vi "Left Motor Control Loop (SubVI).vi"   [LabVIEW 2015]
uses:
  Left Variables.vi
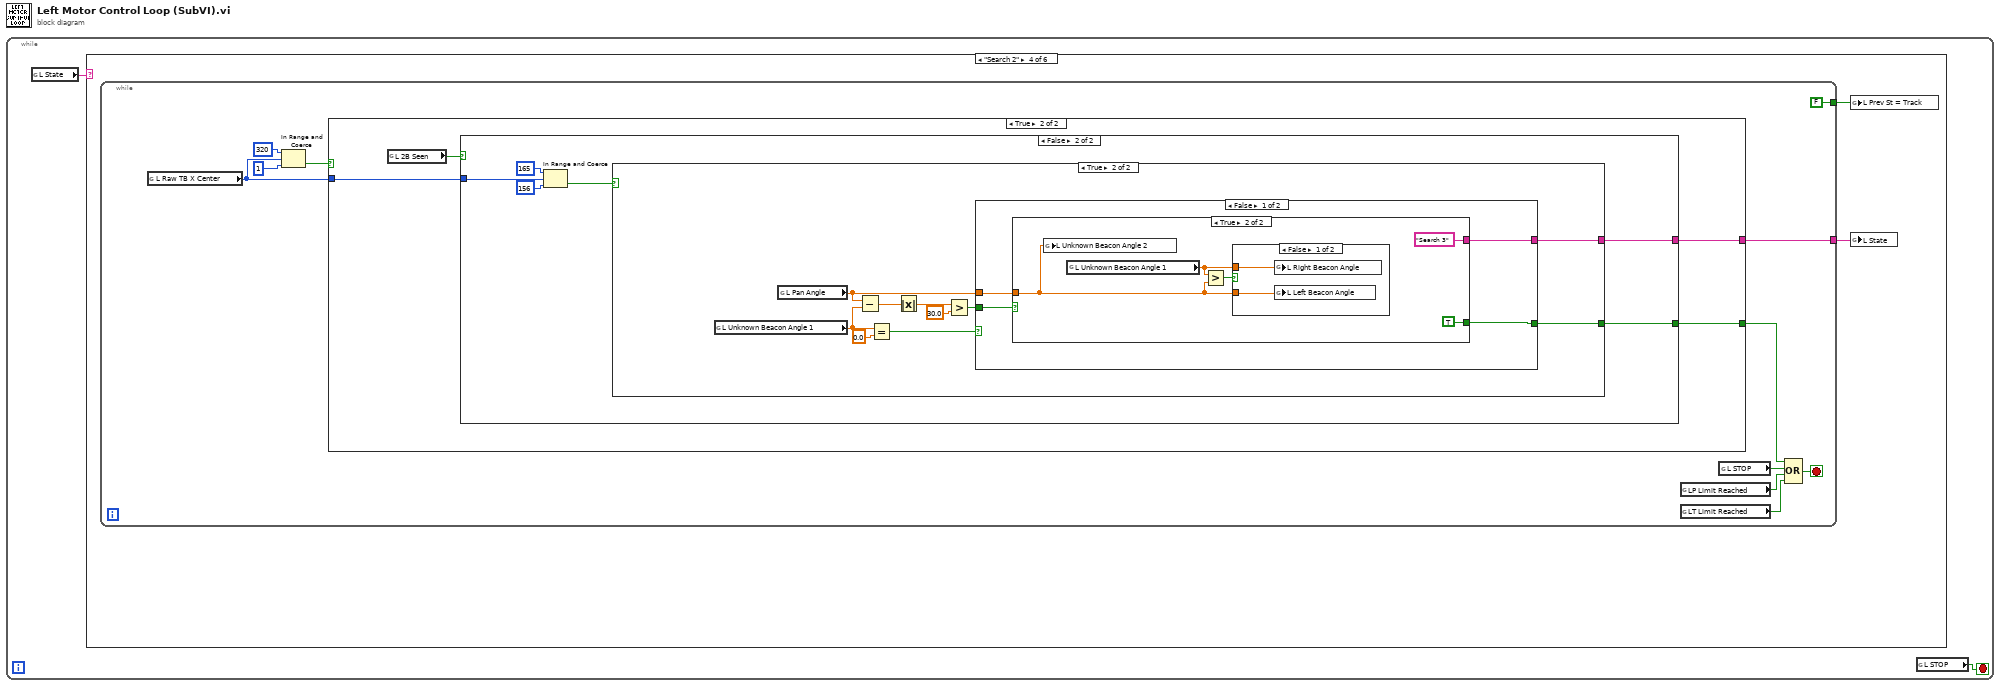
[diagram p0: block diagram]
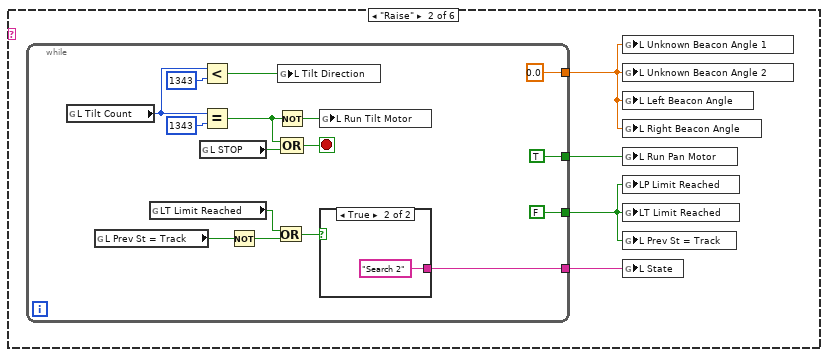
[diagram p3: hidden frame]
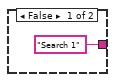
[diagram p4: hidden frame]
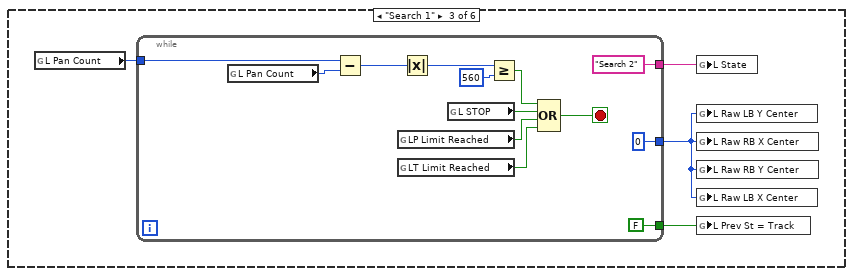
[diagram p5: hidden frame]
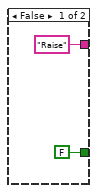
[diagram p6: hidden frame]
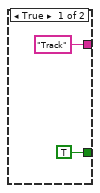
[diagram p7: hidden frame]
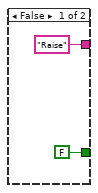
[diagram p8: hidden frame]
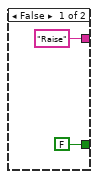
[diagram p9: hidden frame]
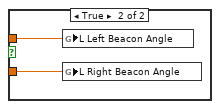
[diagram p10: hidden frame]
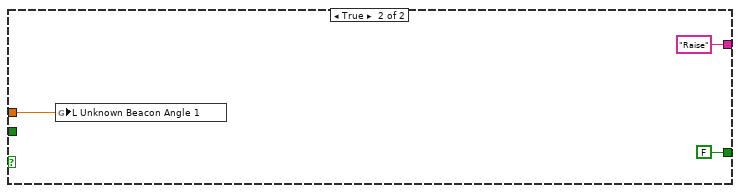
[diagram p11: hidden frame]
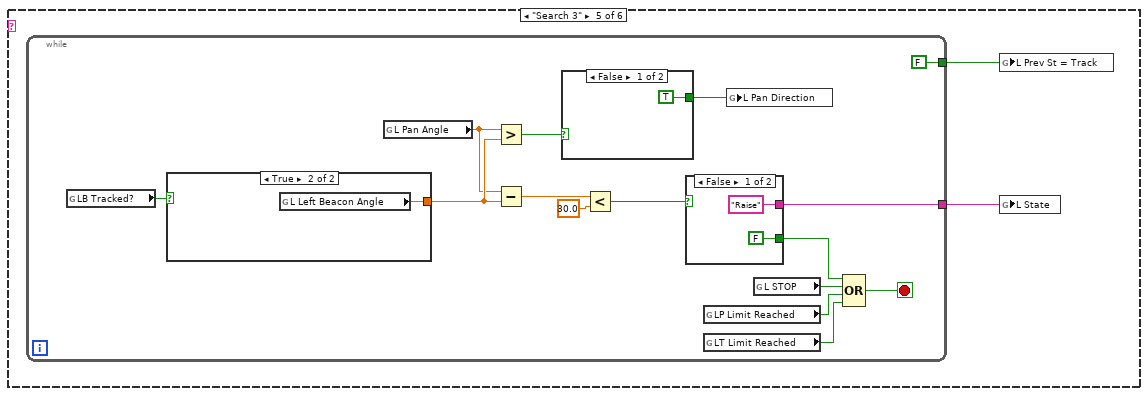
[diagram p12: hidden frame]
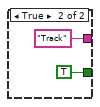
[diagram p13: hidden frame]
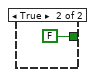
[diagram p14: hidden frame]
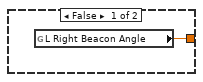
[diagram p15: hidden frame]
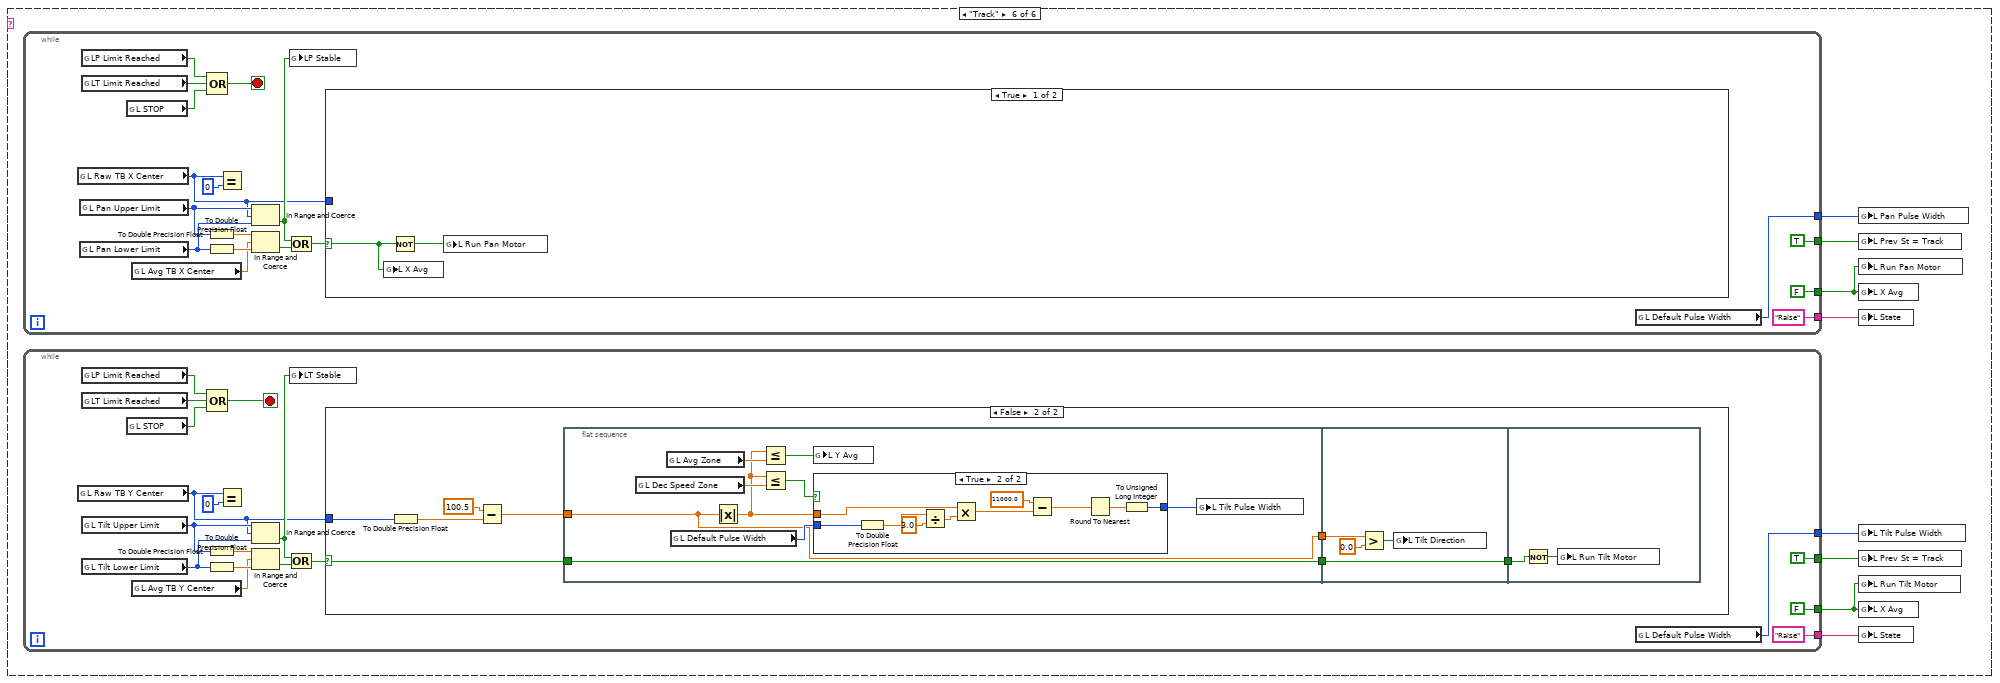
[diagram p16: hidden frame]
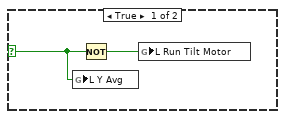
[diagram p17: hidden frame]
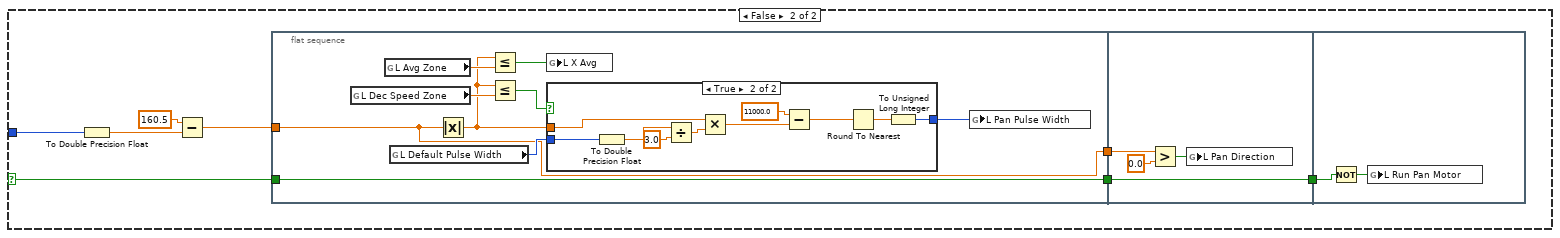
[diagram p19: hidden frame]
diagram:
  n1 = while {
    stop <- w1 stop-if-true
    n2 = global read "Left Variables.vi" "L State"() -> (w2:string)
    n3 = case shown="\"Search 2\"" w2 {
      frame "Null", Default {
      }
      frame "Raise" {
        n4 = while {
          tunnel: [w14] -> w6
          tunnel: [FALSE ("y")] -> w3
          tunnel: [TRUE ("y")] -> w5
          tunnel: [0.0] -> w4
          stop <- w22 stop-if-true
          n5 = global read "Left Variables.vi" "L Tilt Count"() -> (w18:i32)
          n6 = global read "Left Variables.vi" "L Prev St = Track"() -> (w10:bool)
          n7 = global read "Left Variables.vi" "LT Limit Reached"() -> (w8:bool)
          n8 = global read "Left Variables.vi" "L STOP"() -> (w15:bool)
          n9 = Less?(x=w18, y=1343) -> (x < y?=w20:bool)
          n10 = Equal?(x=w18, y=1343) -> (x = y?=w16:bool)
          n11 = Not(x=w10) -> (.not. x?=w9:bool)
          n12 = Or(x=w8, y=w9) -> (x .or. y?=w7:bool)
          n13 = Not(x=w16) -> (.not. x?=w17:bool)
          n14 = global write "Left Variables.vi" "L Tilt Direction"(w20) -> ()
          n15 = Compound Arithmetic op=OR(w16, w15) -> (w22:bool)
          n16 = global write "Left Variables.vi" "L Run Tilt Motor"(w17) -> ()
          n17 = case shown="True" w7 {
            tunnel: ["Search 1" ("L State") "Search 2" ("L State")] -> w14
            frame False {
            }
            frame True {
            }
          }
        }
        n18 = global write "Left Variables.vi" "L Unknown Beacon Angle 1"(w4) -> ()
        n19 = global write "Left Variables.vi" "L Unknown Beacon Angle 2"(w4) -> ()
        n20 = global write "Left Variables.vi" "L Left Beacon Angle"(w4) -> ()
        n21 = global write "Left Variables.vi" "L Right Beacon Angle"(w4) -> ()
        n22 = global write "Left Variables.vi" "L Run Pan Motor"(w5) -> ()
        n23 = global write "Left Variables.vi" "LP Limit Reached"(w3) -> ()
        n24 = global write "Left Variables.vi" "LT Limit Reached"(w3) -> ()
        n25 = global write "Left Variables.vi" "L Prev St = Track"(w3) -> ()
        n26 = global write "Left Variables.vi" "L State"(w6) -> ()
      }
      frame "Search 1" {
        n27 = global read "Left Variables.vi" "L Pan Count"() -> (w27:i32)
        n28 = while {
          tunnel: ["Search 2"] -> w28
          tunnel: w27 -> [w37]
          tunnel: [u16 0] -> w26
          tunnel: [FALSE] -> w25
          stop <- w41 stop-if-true
          n29 = global read "Left Variables.vi" "L Pan Count"() -> (w34:i32)
          n30 = Subtract(x=w37, y=w34) -> (x-y=w36:i32)
          n31 = global read "Left Variables.vi" "LP Limit Reached"() -> (w31:bool)
          n32 = global read "Left Variables.vi" "LT Limit Reached"() -> (w30:bool)
          n33 = Absolute Value(x=w36) -> (abs(x)=w35:i32)
          n34 = global read "Left Variables.vi" "L STOP"() -> (w33:bool)
          n35 = Greater Or Equal?(x=w35, y=560) -> (x >= y?=w38:bool)
          n36 = Compound Arithmetic op=OR(w38, w33, w31, w30) -> (w41:bool)
        }
        n37 = global write "Left Variables.vi" "L State"(w28) -> ()
        n38 = global write "Left Variables.vi" "L Raw LB Y Center"(w26) -> ()
        n39 = global write "Left Variables.vi" "L Raw RB X Center"(w26) -> ()
        n40 = global write "Left Variables.vi" "L Raw RB Y Center"(w26) -> ()
        n41 = global write "Left Variables.vi" "L Raw LB X Center"(w26) -> ()
        n42 = global write "Left Variables.vi" "L Prev St = Track"(w25) -> ()
      }
      frame "Search 2" {
        n43 = while {
          tunnel: [w49] -> w43
          tunnel: [FALSE] -> w42
          stop <- w51 stop-if-true
          n44 = global read "Left Variables.vi" "L Raw TB X Center"() -> (w47:u16)
          n45 = In Range and Coerce(upper limit=u16 320, x=w47, lower limit=u16 1) -> (In Range?=w50:bool)  [unwired: 1 out]
          n46 = case shown="True" w50 {
            tunnel: [FALSE w60] -> w48
            tunnel: ["Raise" w59] -> w49
            tunnel: w47 -> [_ w58]
            frame False {
            }
            frame True {
              n47 = global read "Left Variables.vi" "L 2B Seen"() -> (w57:bool)
              n48 = case shown="False" w57 {
                tunnel: [TRUE w65] -> w60
                tunnel: ["Track" w64] -> w59
                tunnel: w58 -> [_ w63]
                frame True {
                }
                frame False {
                  n49 = In Range and Coerce(upper limit=u16 165, x=w63, lower limit=u16 156) -> (In Range?=w66:bool)  [unwired: 1 out]
                  n50 = case shown="True" w66 {
                    tunnel: [FALSE w73] -> w65
                    tunnel: ["Raise" w72] -> w64
                    frame False {
                    }
                    frame True {
                      n51 = global read "Left Variables.vi" "L Unknown Beacon Angle 1"() -> (w79:dbl)
                      n52 = global read "Left Variables.vi" "L Pan Angle"() -> (w71:dbl)
                      n53 = Subtract(x=w71, y=w79) -> (x-y=w78:dbl)
                      n54 = Equal?(x=w79, y=0.0) -> (x = y?=w75:bool)
                      n55 = Absolute Value(x=w78) -> (abs(x)=w77:dbl)
                      n56 = Greater?(x=w77, y=30.0) -> (0:w74:bool)
                      n57 = case shown="False" w75 {
                        tunnel: w71 -> [w84 w98]
                        tunnel: w74 -> [w83 _]
                        tunnel: [w82 FALSE] -> w73
                        tunnel: [w81 "Raise"] -> w72
                        frame False {
                          n58 = case shown="True" w83 {
                            tunnel: w84 -> [_ w87]
                            tunnel: [FALSE TRUE] -> w82
                            tunnel: ["Raise" "Search 3"] -> w81
                            frame False {
                            }
                            frame True {
                              n59 = global write "Left Variables.vi" "L Unknown Beacon Angle 2"(w87) -> ()
                              n60 = global read "Left Variables.vi" "L Unknown Beacon Angle 1"() -> (w90:dbl)
                              n61 = Greater?(x=w90, y=w87) -> (0:w91:bool)
                              n62 = case shown="False" w91 {
                                tunnel: w90 -> [w93 w95]
                                tunnel: w87 -> [w92 w94]
                                frame False {
                                n63 = global write "Left Variables.vi" "L Right Beacon Angle"(w93) -> ()
                                n64 = global write "Left Variables.vi" "L Left Beacon Angle"(w92) -> ()
                                }
                                frame True {
                                n65 = global write "Left Variables.vi" "L Left Beacon Angle"(w95) -> ()
                                n66 = global write "Left Variables.vi" "L Right Beacon Angle"(w94) -> ()
                                }
                              }
                            }
                          }
                        }
                        frame True {
                          n67 = global write "Left Variables.vi" "L Unknown Beacon Angle 1"(w98) -> ()
                        }
                      }
                    }
                  }
                }
              }
            }
          }
          n68 = global read "Left Variables.vi" "LP Limit Reached"() -> (w46:bool)
          n69 = global read "Left Variables.vi" "LT Limit Reached"() -> (w45:bool)
          n70 = global read "Left Variables.vi" "L STOP"() -> (w52:bool)
          n71 = Compound Arithmetic op=OR(w48, w52, w46, w45) -> (w51:bool)
        }
        n72 = global write "Left Variables.vi" "L Prev St = Track"(w42) -> ()
        n73 = global write "Left Variables.vi" "L State"(w43) -> ()
      }
      frame "Search 3" {
        n74 = while {
          tunnel: [w102] -> w100
          tunnel: [FALSE] -> w99
          stop <- w109 stop-if-true
          n75 = global read "Left Variables.vi" "LB Tracked?"() -> (w108:bool)
          n76 = case shown="True" w108 {
            tunnel: [w122 w123] -> w114
            frame False {
              n77 = global read "Left Variables.vi" "L Right Beacon Angle"() -> (w122:dbl)
            }
            frame True {
              n78 = global read "Left Variables.vi" "L Left Beacon Angle"() -> (w123:dbl)
            }
          }
          n79 = global read "Left Variables.vi" "L Pan Angle"() -> (w106:dbl)
          n80 = Greater?(x=w106, y=w114) -> (0:w115:bool)
          n81 = Subtract(x=w106, y=w114) -> (x-y=w113:dbl)
          n82 = case shown="False" w115 {
            tunnel: [TRUE FALSE] -> w105
            frame False {
            }
            frame True {
            }
          }
          n83 = Less?(x=w113, y=30.0) -> (x < y?=w111:bool)
          n84 = case shown="False" w111 {
            tunnel: ["Raise" "Track"] -> w102
            tunnel: [FALSE TRUE] -> w110
            frame False {
            }
            frame True {
            }
          }
          n85 = global read "Left Variables.vi" "LP Limit Reached"() -> (w104:bool)
          n86 = global read "Left Variables.vi" "LT Limit Reached"() -> (w103:bool)
          n87 = global write "Left Variables.vi" "L Pan Direction"(w105) -> ()
          n88 = global read "Left Variables.vi" "L STOP"() -> (w107:bool)
          n89 = Compound Arithmetic op=OR(w110, w107, w104, w103) -> (w109:bool)
        }
        n90 = global write "Left Variables.vi" "L Prev St = Track"(w99) -> ()
        n91 = global write "Left Variables.vi" "L State"(w100) -> ()
      }
      frame "Track" {
        n92 = while {
          tunnel: ["Raise"] -> w131
          tunnel: [FALSE] -> w129
          tunnel: [TRUE] -> w127
          tunnel: [w186] -> w124
          stop <- w191 stop-if-true
          n93 = global read "Left Variables.vi" "L Raw TB X Center"() -> (w189:u16)
          n94 = global read "Left Variables.vi" "L Pan Upper Limit"() -> (w199:u16)
          n95 = global read "Left Variables.vi" "L Pan Lower Limit"() -> (w198:u16)
          n96 = global read "Left Variables.vi" "LP Limit Reached"() -> (w192:bool)
          n97 = global read "Left Variables.vi" "LT Limit Reached"() -> (w194:bool)
          n98 = global read "Left Variables.vi" "L STOP"() -> (w193:bool)
          n99 = global read "Left Variables.vi" "L Avg TB X Center"() -> (w195:dbl)
          n100 = Compound Arithmetic op=OR(w192, w194, w193) -> (w191:bool)
          n101 = To Double Precision Float(number=w199) -> (double precision float=w201:dbl)
          n102 = To Double Precision Float(number=w198) -> (double precision float=w200:dbl)
          n103 = Equal?(x=w189, y=u16 0) -> ()  [unwired: 1 out]
          n104 = In Range and Coerce(upper limit=w199, x=w189, lower limit=w198) -> (In Range?=w197:bool)  [unwired: 1 out]
          n105 = In Range and Coerce(upper limit=w201, x=w195, lower limit=w200) -> (In Range?=w196:bool)  [unwired: 1 out]
          n106 = global write "Left Variables.vi" "LP Stable"(w197) -> ()
          n107 = Compound Arithmetic op=OR(w197, w196) -> (w202:bool)
          n108 = case shown="True" w202 {
            selector: w202 -> [w204 w208]
            tunnel: w189 -> [_ w213]
            frame True {
              n109 = global write "Left Variables.vi" "L X Avg"(w204) -> ()
              n110 = Not(x=w204) -> (.not. x?=w205:bool)
              n111 = global write "Left Variables.vi" "L Run Pan Motor"(w205) -> ()
            }
            frame False {
              n112 = To Double Precision Float(number=w213) -> (double precision float=w211:dbl)
              n113 = Subtract(x=160.5, y=w211) -> (x-y=w210:dbl)
              n114 = flat-sequence {
                tunnel: w210 -> [w215]
                tunnel: [w215] -> w209
                tunnel: w208 -> [w214]
                tunnel: [w214] -> w207
                tunnel: w209 -> [w235]
                tunnel: w207 -> [w234]
                tunnel: [w234] -> w206
                tunnel: w206 -> [w238]
                frame #0 {
                  n115 = global read "Left Variables.vi" "L Dec Speed Zone"() -> (w220:dbl)
                  n116 = global read "Left Variables.vi" "L Avg Zone"() -> (w219:dbl)
                  n117 = global read "Left Variables.vi" "L Default Pulse Width"() -> (w221:u32)
                  n118 = Absolute Value(x=w215) -> (abs(x)=w217:dbl)
                  n119 = Less Or Equal?(x=w217, y=w219) -> (x <= y?=w218:bool)
                  n120 = Less Or Equal?(x=w217, y=w220) -> (x <= y?=w222:bool)
                  n121 = global write "Left Variables.vi" "L X Avg"(w218) -> ()
                  n122 = case shown="True" w222 {
                    tunnel: w221 -> [w223 w233]
                    tunnel: [w223 w226] -> w216
                    tunnel: w217 -> [_ w224]
                    frame False {
                    }
                    frame True {
                      n123 = To Double Precision Float(number=w233) -> (double precision float=w225:dbl)
                      n124 = Divide(x=w225, y=3.0) -> (x/y=w230:dbl)
                      n125 = Multiply(x=w224, y=w230) -> (x*y=w229:dbl)
                      n126 = Subtract(x=11000.0, y=w229) -> (x-y=w228:dbl)
                      n127 = Round To Nearest(number=w228) -> (nearest integer value=w227:dbl)
                      n128 = To Unsigned Long Integer(number=w227) -> (unsigned 32bit integer=w226:u32)
                    }
                  }
                  n129 = global write "Left Variables.vi" "L Pan Pulse Width"(w216) -> ()
                }
                frame #1 {
                  n130 = Greater?(x=w235, y=0.0) -> (0:w237:bool)
                  n131 = global write "Left Variables.vi" "L Pan Direction"(w237) -> ()
                }
                frame #2 {
                  n132 = Not(x=w238) -> (.not. x?=w239:bool)
                  n133 = global write "Left Variables.vi" "L Run Pan Motor"(w239) -> ()
                }
              }
            }
          }
          n134 = global read "Left Variables.vi" "L Default Pulse Width"() -> (w186:u32)
        }
        n135 = while {
          tunnel: ["Raise"] -> w130
          tunnel: [FALSE] -> w128
          tunnel: [TRUE] -> w126
          tunnel: [w132] -> w125
          stop <- w149 stop-if-true
          n136 = global read "Left Variables.vi" "L Raw TB Y Center"() -> (w136:u16)
          n137 = global read "Left Variables.vi" "LP Limit Reached"() -> (w135:bool)
          n138 = global read "Left Variables.vi" "LT Limit Reached"() -> (w148:bool)
          n139 = global read "Left Variables.vi" "L Tilt Upper Limit"() -> (w143:u16)
          n140 = global read "Left Variables.vi" "L Tilt Lower Limit"() -> (w142:u16)
          n141 = global read "Left Variables.vi" "L STOP"() -> (w146:bool)
          n142 = global read "Left Variables.vi" "L Avg TB Y Center"() -> (w138:dbl)
          n143 = Compound Arithmetic op=OR(w135, w148, w146) -> (w149:bool)
          n144 = To Double Precision Float(number=w143) -> (double precision float=w145:dbl)
          n145 = To Double Precision Float(number=w142) -> (double precision float=w144:dbl)
          n146 = Equal?(x=w136, y=u16 0) -> ()  [unwired: 1 out]
          n147 = In Range and Coerce(upper limit=w143, x=w136, lower limit=w142) -> (In Range?=w141:bool)  [unwired: 1 out]
          n148 = In Range and Coerce(upper limit=w145, x=w138, lower limit=w144) -> (In Range?=w140:bool)  [unwired: 1 out]
          n149 = global write "Left Variables.vi" "LT Stable"(w141) -> ()
          n150 = Compound Arithmetic op=OR(w141, w140) -> (w139:bool)
          n151 = case shown="False" w139 {
            selector: w139 -> [w150 w152]
            tunnel: w136 -> [_ w159]
            frame True {
              n152 = global write "Left Variables.vi" "L Y Avg"(w150) -> ()
              n153 = Not(x=w150) -> (.not. x?=w151:bool)
              n154 = global write "Left Variables.vi" "L Run Tilt Motor"(w151) -> ()
            }
            frame False {
              n155 = To Double Precision Float(number=w159) -> (double precision float=w157:dbl)
              n156 = Subtract(x=100.5, y=w157) -> (x-y=w156:dbl)
              n157 = flat-sequence {
                tunnel: w156 -> [w161]
                tunnel: [w161] -> w155
                tunnel: [w160] -> w153
                tunnel: w152 -> [w160]
                tunnel: w155 -> [w181]
                tunnel: [w180] -> w154
                tunnel: w153 -> [w180]
                tunnel: w154 -> [w184]
                frame #0 {
                  n158 = global read "Left Variables.vi" "L Dec Speed Zone"() -> (w167:dbl)
                  n159 = global read "Left Variables.vi" "L Avg Zone"() -> (w165:dbl)
                  n160 = global read "Left Variables.vi" "L Default Pulse Width"() -> (w166:u32)
                  n161 = Absolute Value(x=w161) -> (abs(x)=w163:dbl)
                  n162 = Less Or Equal?(x=w163, y=w165) -> (x <= y?=w164:bool)
                  n163 = Less Or Equal?(x=w163, y=w167) -> (x <= y?=w168:bool)
                  n164 = global write "Left Variables.vi" "L Y Avg"(w164) -> ()
                  n165 = case shown="True" w168 {
                    tunnel: w166 -> [w169 w173]
                    tunnel: [w169 w172] -> w162
                    tunnel: w163 -> [_ w170]
                    frame False {
                    }
                    frame True {
                      n166 = To Double Precision Float(number=w173) -> (double precision float=w171:dbl)
                      n167 = Divide(x=w171, y=3.0) -> (x/y=w176:dbl)
                      n168 = Multiply(x=w170, y=w176) -> (x*y=w177:dbl)
                      n169 = Subtract(x=11000.0, y=w177) -> (x-y=w178:dbl)
                      n170 = Round To Nearest(number=w178) -> (nearest integer value=w179:dbl)
                      n171 = To Unsigned Long Integer(number=w179) -> (unsigned 32bit integer=w172:u32)
                    }
                  }
                  n172 = global write "Left Variables.vi" "L Tilt Pulse Width"(w162) -> ()
                }
                frame #1 {
                  n173 = Greater?(x=w181, y=0.0) -> (0:w183:bool)
                  n174 = global write "Left Variables.vi" "L Tilt Direction"(w183) -> ()
                }
                frame #2 {
                  n175 = Not(x=w184) -> (.not. x?=w185:bool)
                  n176 = global write "Left Variables.vi" "L Run Tilt Motor"(w185) -> ()
                }
              }
            }
          }
          n177 = global read "Left Variables.vi" "L Default Pulse Width"() -> (w132:u32)
        }
        n178 = global write "Left Variables.vi" "L Pan Pulse Width"(w124) -> ()
        n179 = global write "Left Variables.vi" "L Prev St = Track"(w127) -> ()
        n180 = global write "Left Variables.vi" "L Run Pan Motor"(w129) -> ()
        n181 = global write "Left Variables.vi" "L X Avg"(w129) -> ()
        n182 = global write "Left Variables.vi" "L State"(w131) -> ()
        n183 = global write "Left Variables.vi" "L Tilt Pulse Width"(w125) -> ()
        n184 = global write "Left Variables.vi" "L Prev St = Track"(w126) -> ()
        n185 = global write "Left Variables.vi" "L Run Tilt Motor"(w128) -> ()
        n186 = global write "Left Variables.vi" "L X Avg"(w128) -> ()
        n187 = global write "Left Variables.vi" "L State"(w130) -> ()
      }
    }
    n188 = global read "Left Variables.vi" "L STOP"() -> (w1:bool)
  }
